vi "Too Close to Nav Borders.vi"() -> (0 "Too Close?":bool, 1 "Bearing to Avoid":dbl)   [LabVIEW 2009]
panel:
  in  "Threshold (meters)":dbl=3.0
  out "Longitude Threshold":dbl
  out "Latitude Threshold":dbl
  in  "South Latitude":dbl=2560.73698378 format="%#_14g"
  in  "North Latitude":dbl=2560.7721892 format="%#_14g"
  in  "East Longitude":dbl=4991.69493291 format="%#_14g"
  in  "West Longitude":dbl=4991.73537269 format="%#_14g"
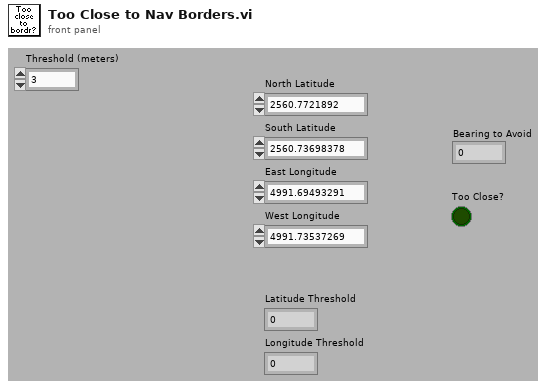
[diagram p1: front panel]
types:
  T1 = typedef "GPS Data.ctl" = cluster{"Latitude":dbl, "Longitude":dbl}
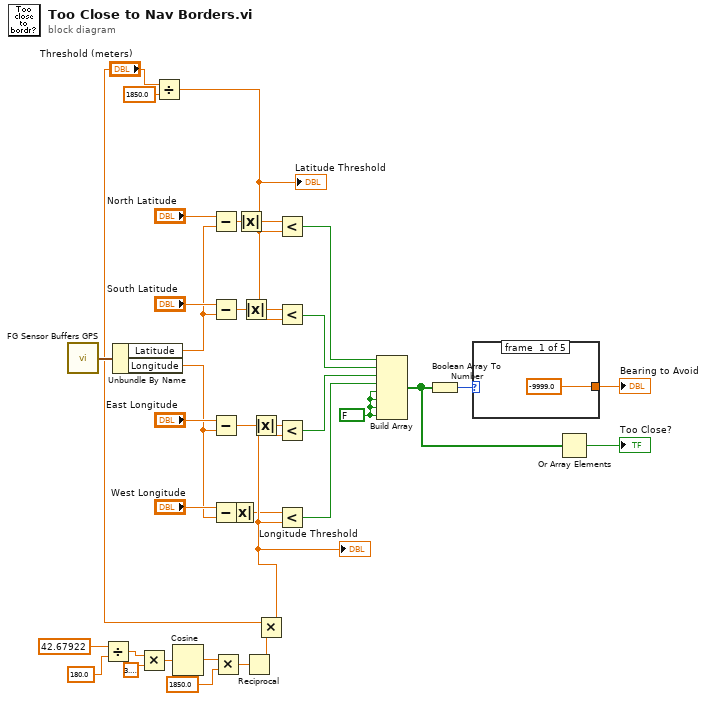
[diagram p0: block diagram]
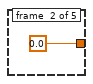
[diagram p2: hidden frame]
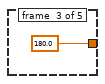
[diagram p3: hidden frame]
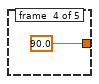
[diagram p4: hidden frame]
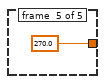
[diagram p5: hidden frame]
diagram:
  w22 = FALSE ("x < y?")
  n1 = call "FG Sensor Buffers GPS.vi"() -> ("GPS Buffer out"=w33:T1)  [unwired: 2 in]
  n2 = Divide(x=42.67922 ("y"), y=180.0) -> (x/y=w13:dbl)
  n3 = Unbundle By Name(w33) -> ("Latitude"=w32:dbl, "Longitude"=w31:dbl)
  n4 = Multiply(x=w13, y=3.141592653589793) -> (x*y=w11:dbl)
  n5 = Divide(x="Threshold (meters)", y=1850.0) -> (x/y=w16:dbl)
  "Latitude Threshold" <- w16
  n6 = Cosine(x=w11) -> (cos(x)=w10:dbl)
  n7 = Subtract(x="North Latitude", y=w32) -> (x-y=w30:dbl)
  n8 = Subtract(x="South Latitude", y=w32) -> (x-y=w29:dbl)
  n9 = Subtract(x="East Longitude", y=w31) -> (x-y=w28:dbl)
  n10 = Subtract(x="West Longitude", y=w31) -> (x-y=w27:dbl)
  n11 = Multiply(x=w10, y=1850.0) -> (x*y=w8:dbl)
  n12 = Absolute Value(x=w27) -> (abs(x)=w1:dbl)
  n13 = Absolute Value(x=w30) -> (abs(x)=w4:dbl)
  n14 = Absolute Value(x=w29) -> (abs(x)=w3:dbl)
  n15 = Reciprocal(x=w8) -> (1/x=w7:dbl)
  n16 = Absolute Value(x=w28) -> (abs(x)=w2:dbl)
  n17 = Multiply(x="Threshold (meters)", y=w7) -> (x*y=w6:dbl)
  "Longitude Threshold" <- w6
  n18 = Less?(x=w4, y=w16) -> (x < y?=w26:bool)
  n19 = Less?(x=w3, y=w16) -> (x < y?=w25:bool)
  n20 = Less?(x=w2, y=w6) -> (x < y?=w24:bool)
  n21 = Less?(x=w1, y=w6) -> (x < y?=w23:bool)
  n22 = Build Array(w26, w25, w24, w23, w22, w22, w22, w22) -> (w20:bool[])
  n23 = Boolean Array To Number(Boolean array=w20) -> (number=w19:u32)
  n24 = case shown="1000" w19 {
    tunnel: [-9999.0 ("Latitude Threshold") 0.0 ("Latitude Threshold") 180.0 ("Latitude Threshold") 90.0 ("Latitude Threshold") 270.0 ("Latitude Threshold")] -> w18
    frame #0 {
    }
    frame #1 {
    }
    frame #2 {
    }
    frame #3 {
    }
    frame #4 {
    }
  }
  "Bearing to Avoid" <- w18
  n25 = Or Array Elements(Boolean array=w20) -> (logical OR=→"Too Close?":bool)
